vi "aryapp.vi"() -> ()   [LabVIEW 2022 SP3]
panel:
  in  "下":bool
  in  "Stop":bool
  in  "列":dbl
  in  "行":dbl
  out "Array":bool[][](array[boolean])=[[TRUE, TRUE, TRUE], [TRUE, FALSE, TRUE], [TRUE, TRUE, TRUE]]
  out "Boolean":bool=TRUE
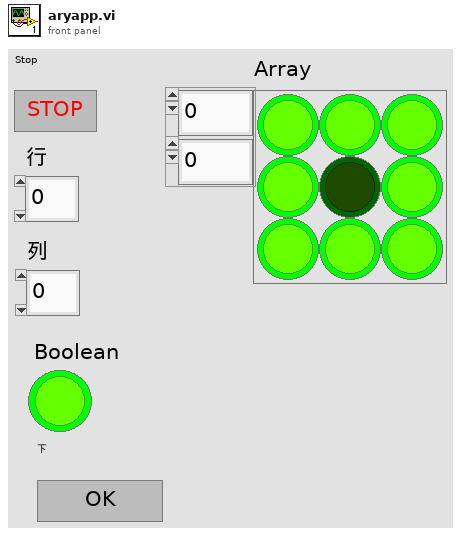
[diagram p1: front panel]
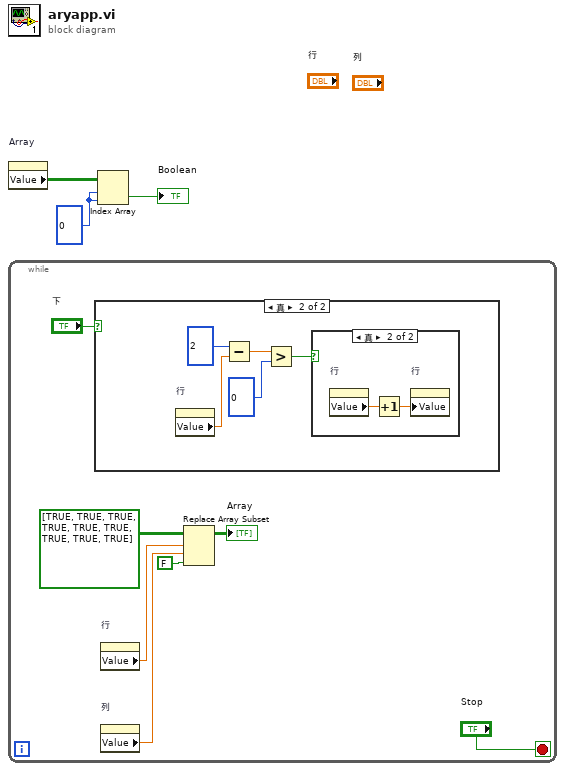
[diagram p0: block diagram]
diagram:
  w3 = 0
  n1 = property on="Array" class="Arr (严格)"() -> ("Value"=w1:bool[][])  [unwired: 2 in, 2 out]
  n2 = while {
    stop <- "Stop" stop-if-true
    n3 = case shown="真" "下" {
      frame False {
      }
      frame True {
        n4 = property on="行" class="DigNum (严格)"() -> ("Value"=w11:dbl)  [unwired: 2 in, 2 out]
        n5 = Subtract(x=2, y=w11) -> (x-y=w13:dbl)
        n6 = Greater?(x=w13, y=0) -> (0:w14:bool)
        n7 = case shown="真" w14 {
          frame False {
          }
          frame True {
            n8 = property on="行" class="DigNum (严格)"() -> ("Value"=w17:dbl)  [unwired: 2 in, 2 out]
            n9 = Increment(x=w17) -> (x+1=w16:dbl)
            n10 = property on="行" class="DigNum (严格)"("Value"=w16) -> ()  [unwired: 2 in, 2 out]
          }
        }
      }
    }
    n11 = property on="行" class="DigNum (严格)"() -> ("Value"=w7:dbl)  [unwired: 2 in, 2 out]
    n12 = property on="列" class="DigNum (严格)"() -> ("Value"=w6:dbl)  [unwired: 2 in, 2 out]
    n13 = Replace Array Subset(array=bool[][] [[TRUE, TRUE, TRUE], [TRUE, TRUE, TRUE], [TRUE, TRUE, TRUE]], new element=FALSE, index (row)=w7, index (col)=w6) -> (→"Array":bool[][])
  }
  n14 = Index Array(array=w1, index (row)=w3, index (col)=w3) -> (element=→"Boolean":bool)
